vi "Format Error Core.vi"(0 "error handler in":refnum<class "TLB` Error Handler.lvclass">) -> (4 "error handler out":refnum<class "TLB` Error Handler.lvclass">, 8 "source text":string)   [LabVIEW 2015, in "TLB` Template.lvlib" / "TLB` Error Handler.lvclass"]
uses:
  TLB` Error Handler.lvclass
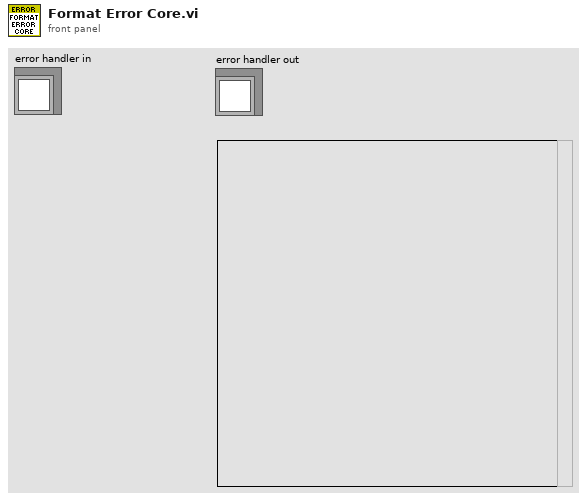
[diagram p1: front panel]
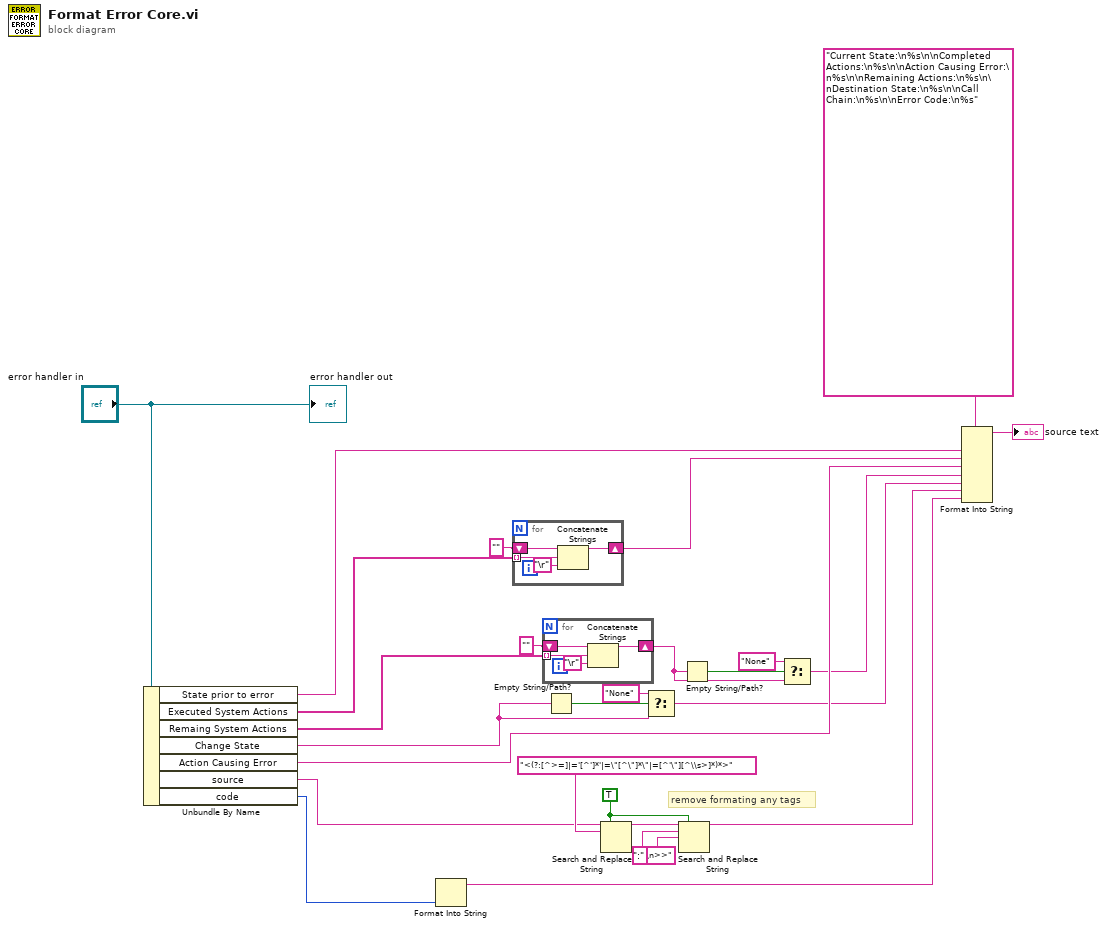
[diagram p0: block diagram]
diagram:
  w7 = TRUE ("replace all? (F)")
  # "remove formating any tags"
  n1 = Unbundle By Name("error handler in") -> ("State prior to error"=w10:string, "Executed System Actions"=w20:string[], "Remaing System Actions"=w21:string[], "Change State"=w22:string, "Action Causing Error"=w3:string, "source"=w8:string, "code"=w12:i32)
  n2 = Format Into String(w12) -> (resulting string=w11:string)  [unwired: 3 in, 1 out]
  n3 = for {
    tunnel: w20 -> [w30] mode=indexing
    shift-right: [w28] -> w13
    shift-left: "" -> [w31]
    n4 = Concatenate Strings(w31, w30, "\r") -> (w28:string)
  }
  n5 = for {
    tunnel: w21 -> [w34] mode=indexing
    shift-right: [w32] -> w25
    shift-left: "" -> [w35]
    n6 = Concatenate Strings(w35, w34, "\r") -> (w32:string)
  }
  n7 = Empty String/Path?(string/path=w22) -> (empty?=w23:bool)
  n8 = Search and Replace String(replace all?=w7, input string=w8, search string="<(?:[^>=]|='[^']*'|=\"[^\"]*\"|=[^'\"][^\\s>]*)*>") -> (result string=w9:string)  [unwired: 5 in, 3 out]
  n9 = Select(t="None", s=w23, f=w22) -> (s? t:f=w1:string)
  n10 = Search and Replace String(replace all?=w7, input string=w9, search string=":", replace string="\n>>" ("replace string (\"\")")) -> (result string=w4:string)  [unwired: 4 in, 3 out]
  n11 = Empty String/Path?(string/path=w25) -> (empty?=w24:bool)
  n12 = Select(t="None", s=w24, f=w25) -> (s? t:f=w2:string)
  n13 = Format Into String(format string="Current State:\n%s\n\nCompleted Actions:\n%s\n\nAction Causing Error:\n%s\n\nRemaining Actions:\n%s\n\nDestination State:\n%s\n\nCall Chain:\n%s\n\nError Code:\n%s", w10, w13, w3, w2, w1, w4, w11) -> (resulting string=→"source text":string)  [unwired: 2 in, 1 out]
  "error handler out" <- "error handler in"
